vi "Update_PictureBox.vi"(9 "Tip Strip":string, 10 "Picture Path":path, 11 "Picture Box in":refnum<vi>) -> (0 "error out":errorcluster, 1 "Y-Axis ratio (correction factor)":dbl, 2 "X-Axis ratio":dbl, 3 "Draw Area Size":T1, 5 "Picture's path string (out)":string)   [LabVIEW 2017]
uses:
  <vilib>/Utility/miscctls.llb/LVBoundsTypeDef.ctl
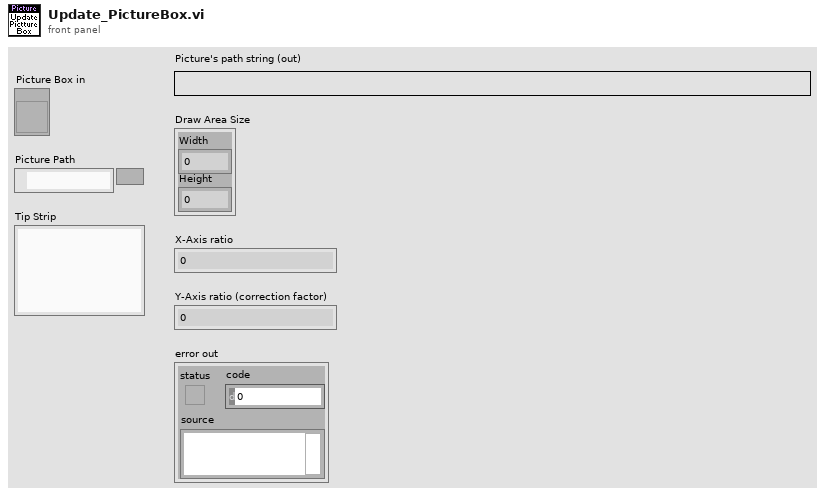
[diagram p1: front panel]
types:
  T1 = typedef "LVBoundsTypeDef.ctl" = cluster{"Width":u32, "Height":u32}
  T2 = typedef "imagedata.ctl" = cluster{"image type":i32, "image depth":i32, "image":u8[], "mask":u8[], "colors":u32[], "Rectangle":cluster{"left":i16, "top":i16, "right":i16, "bottom":i16}}
  T3 = typedef "LVPointTypeDef.ctl" = cluster{"Horizontal":i16, "Vertical":i16}
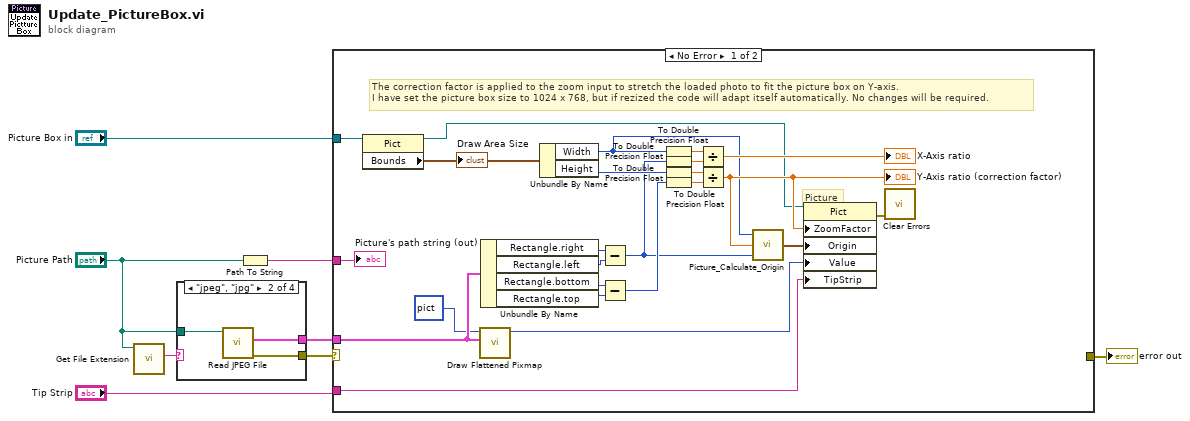
[diagram p0: block diagram]
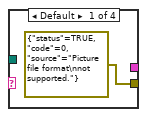
[diagram p2: hidden frame]
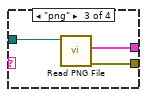
[diagram p3: hidden frame]
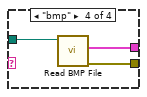
[diagram p4: hidden frame]
diagram:
  n1 = call <vilib>:"Get File Extension.vi"("file"="Picture Path") -> ("lowercase file extension"=w1:string)  [unwired: 6 in, 4 out]
  n2 = case shown="\"jpeg\", \"jpg\"" w1 {
    tunnel: [errorcluster {"status"=TRUE, "code"=0, "source"="Picture file format\nnot supported."} ("error out") w12 w13 w16] -> w5
    tunnel: [_ w11 w14 w17] -> w3
    tunnel: "Picture Path" -> [_ w10 w15 w18]
    frame Default {
    }
    frame "jpeg", "jpg" {
      n3 = call <vilib>:"Read JPEG File.vi"("path to JPEG file"=w10) -> ("error out"=w12:errorcluster, "image data"=w11:T2)  [unwired: 1 in, 8 out]
    }
    frame "png" {
      n4 = call <vilib>:"Read PNG File.vi"("path to PNG file"=w15) -> ("error out"=w13:errorcluster, "image data"=w14:T2)  [unwired: 8 in, 1 out]
    }
    frame "bmp" {
      n5 = call <vilib>:"Read BMP File.vi"("path to BMP file"=w18) -> ("error out"=w16:errorcluster, "image data"=w17:T2)  [unwired: 8 in, 1 out]
    }
  }
  n6 = Path To String(path="Picture Path") -> (string=w6:string)
  n7 = case shown="No Error" w5 {
    selector: w5 -> [_ w43]
    tunnel: w3 -> [w38 _]
    tunnel: "Tip Strip" -> [w29 _]
    tunnel: "Picture Box in" -> [w20 _]
    tunnel: w6 -> [w28 _]
    tunnel: [_ w43] -> w7
    frame No Error {
      # "Picture"
      # "The correction factor is applied to the zoom input to stretch the loaded photo to fit the picture box on Y-axis.\nI have set the picture box size to 1024 x 768, but if rezized the code will adapt itself automatically. No changes will be required."
      n8 = property on="Property Node" class="Pict"(reference=w20) -> (reference out=w19:refnum<vi>, "Bounds"=w35:T1)  [unwired: 1 in, 1 out]
      "Draw Area Size" <- w35
      n9 = call <vilib>:"Draw Flattened Pixmap.vi"("image data"=w38, "picture"=picture data[5B] ("Picture")) -> ("new picture"=w25:picture)  [unwired: 7 out]
      n10 = Unbundle By Name(w38) -> ("Rectangle.right"=w41:i16, "Rectangle.left"=w42:i16, "Rectangle.bottom"=w39:i16, "Rectangle.top"=w40:i16)
      n11 = Unbundle By Name(w35) -> ("Width"=w21:u32, "Height"=w34:u32)
      n12 = Subtract(x=w41, y=w42) -> (x-y=w23:i16)
      n13 = Subtract(x=w39, y=w40) -> (x-y=w24:i16)
      n14 = To Double Precision Float(number=w21) -> (double precision float=w33:dbl)
      n15 = To Double Precision Float(number=w23) -> (double precision float=w32:dbl)
      n16 = To Double Precision Float(number=w34) -> (double precision float=w31:dbl)
      n17 = To Double Precision Float(number=w24) -> (double precision float=w30:dbl)
      n18 = Divide(x=w33, y=w32) -> (x/y=→"X-Axis ratio":dbl)
      n19 = Divide(x=w31, y=w30) -> (x/y=w22:dbl)
      "Y-Axis ratio (correction factor)" <- w22
      n20 = call "Picture_Calculate_Origin.vi"("Loaded Picture Width (in pixels)"=w23, "Y-Axis ratio (correction factor)"=w22, "PictureBox.DrawAreaSize.Width"=w21) -> ("Origin"=w26:T3)
      n21 = property on="Property Node" class="Pict"(reference=w19, "ZoomFactor"=w22, "Origin"=w26, "Value"=w25, "TipStrip"=w29) -> (error out=w36:errorcluster)  [unwired: 1 in, 1 out]
      n22 = call <vilib>:"Clear Errors.vi"("error in (no error)"=w36) -> ()  [unwired: 5 in, 2 out]
      "Picture's path string (out)" <- w28
    }
    frame Error {
    }
  }
  "error out" <- w7
